vi "Measure Zero Span.vi"(8 "error in (no error)":errorcluster, 10 "Center Frequency (Hz)":dbl=1000000000.0 format="%_9p", 11 "SpecA_MXA.lvclass":refnum<class "SpecA_MXA.lvclass">) -> (0 "error out":errorcluster, 1 "Marker Position (Delta Hz)":dbl format="%#_6p", 2 "Marker Amplitude (dBm)":dbl format="%#_6f", 3 "SpecA_MXA.lvclass":refnum<class "SpecA_MXA.lvclass">)   [LabVIEW 2014, in "SpecA_MXA.lvclass"]
uses:
  SpecA_MXA.lvclass
  SpecA_MXA.lvclass/SpecA_MXA.ctl
  <instrlib>/Agilent MXA Series/Public/Configure/Configure Frequency (Center Span).vi
  <instrlib>/Agilent MXA Series/Agilent MXA Series.lvlib
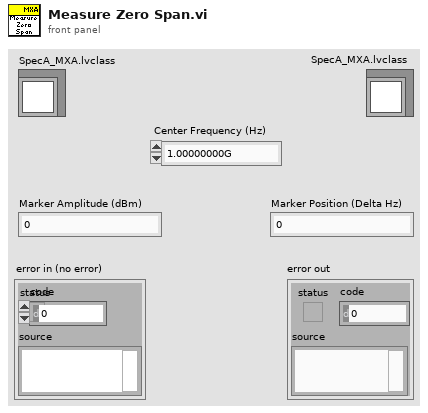
[diagram p1: front panel]
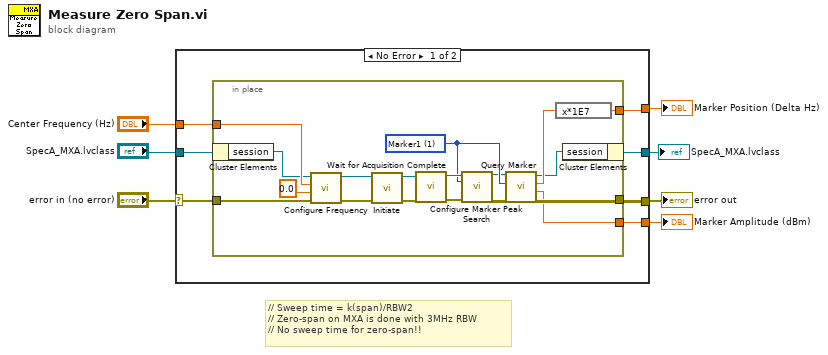
[diagram p0: block diagram]
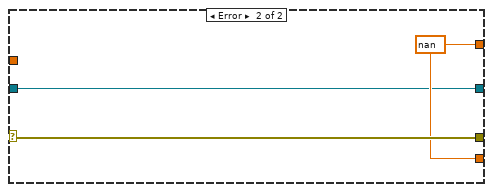
[diagram p2: hidden frame]
diagram:
  # "// Sweep time = k(span)/RBW2\n// Zero-span on MXA is done with 3MHz RBW\n// No sweep time for zero-span!!"
  n1 = case shown="No Error" "error in (no error)" {
    selector: "error in (no error)" -> [w10 w35]
    tunnel: [w13 w35] -> w6
    tunnel: "Center Frequency (Hz)" -> [w14 _]
    tunnel: [w11 w34] -> w4
    tunnel: [w12 w34] -> w3
    tunnel: "SpecA_MXA.lvclass" -> [w9 w33]
    tunnel: [w8 w33] -> w1
    frame No Error {
      n2 = in-place {
        in-place-border: w14 -> [w31]
        in-place-border: [w15] -> w13
        in-place-border: [w30] -> w12
        in-place-border: [w28] -> w11
        in-place-border: w10 -> [w25]
        w23 = 1 items=["Marker1"=1, "Marker2"=2, "Marker3"=3, "Marker4"=4, "Marker5"=5, "Marker6"=6, "Marker7"=7, "Marker8"=8, "Marker9"=9, "Marker10"=10, "Marker11"=11, "Marker12"=12] ("Active Marker (1: Marker1)")
        n3 = in-place-cluster #1(w9) -> ("session"=w22:refnum<visa-resource-name>)
        n4 = call-poly <instrlib>:"Configure Frequency.vi"("error in (no error)"=w25, "Span (2.65E+10 Hz)"=0.0, "Center Frequency (1.325E+10 Hz)"=w31, "VISA resource name"=w22) -> ("error out"=w20:errorcluster, "VISA resource name out"=w26:refnum<visa-resource-name>)  [unwired: 6 in]
        n5 = call <instrlib>:"Initiate.vi"("error in (no error)"=w20, "VISA resource name"=w26) -> ("error out"=w19:errorcluster, "VISA resource name out"=w27:refnum<visa-resource-name>)  [unwired: 8 in]
        n6 = call <instrlib>:"Wait for Acquisition Complete.vi"("error in (no error)"=w19, "VISA resource name"=w27) -> ("error out"=w18:errorcluster, "VISA resource name out"=w24:refnum<visa-resource-name>)  [unwired: 8 in]
        n7 = call <instrlib>:"Configure Marker Peak Search.vi"("VISA resource name"=w24, "Active Marker (1: Marker1)"=w23, "error in (no error)"=w18) -> ("VISA resource name out"=w16:refnum<visa-resource-name>, "error out"=w17:errorcluster)  [unwired: 11 in]
        n8 = call <instrlib>:"Query Marker.vi"("error in (no error)"=w17, "Active Marker (1: Marker1)"=w23, "VISA resource name"=w16) -> ("error out"=w15:errorcluster, "Marker Amplitude"=w30:dbl, "Marker Position"=w29:dbl, "VISA resource name out"=w21:refnum<visa-resource-name>)  [unwired: 5 in]
        n9 = expression code="x*1E7" ("us to s")(w29) -> (w28:dbl)
        n10 = in-place-cluster #1("session"=w21) -> (w8:refnum<class "SpecA_MXA.lvclass">)
      }
    }
    frame Error {
      w34 = nan ("Marker Position")
    }
  }
  "error out" <- w6
  "Marker Position (Delta Hz)" <- w4
  "Marker Amplitude (dBm)" <- w3
  "SpecA_MXA.lvclass" <- w1
